vi "results graphing.vi"(0 "set to view":u32) -> (1 "N Meas":i32, 2 "Temperature":dbl, 3 "RC Fit":T4, 4 "RC Graph":waveform(dbl), 8 "results out":T3[](array[typedef]), 11 "N waves":i32 caption="Number of Waveforms", 12 "N done":i32 caption="Number Complete", 13 "meas":T1={"wvfm params"={"Num of avg"=100, "Num points"=1000, "Meas rate (Hz)"=100000.0}, "avg"={"t0"=timestamp(0 s since 1904-01-01), "dt"=1.0, "Y"=[]}, "raw wvfms"=[], "progress"={"avg done"=FALSE, "meas index"=0, "N waves"=0}, "t (s)"=0.0}, 14 "raw wvfms":waveform(dbl)[](array[waveform]), 15 "C vs T graph":cluster{dbl[], dbl[]})   [LabVIEW 2019]
doc: "This is a Bug C(T) subVI.\n\nIt extracts a variety of data from the results for presentation in the monitor loop.\n\nPaul K Dixon\nP3600\nCSUSB Physics"
uses:
  typedefs/result.ctl
  typedefs/cap fit params.ctl
  typedefs/measurement.ctl
  typedefs/wvfm acq params.ctl
  globals/Bug globals.vi
panel:
  out "result":T3={"Temp (C)"=0.0, "RC Fit"={"Resistance (Ohms)"=100000.0, "Est Time constant (s)"=0.0, "Est Capacitance (F)"=0.0}, "wave"={"t0"=timestamp(0 s since 1904-01-01), "dt"=1.0, "Y"=[]}, "Time (s)"=0.0}
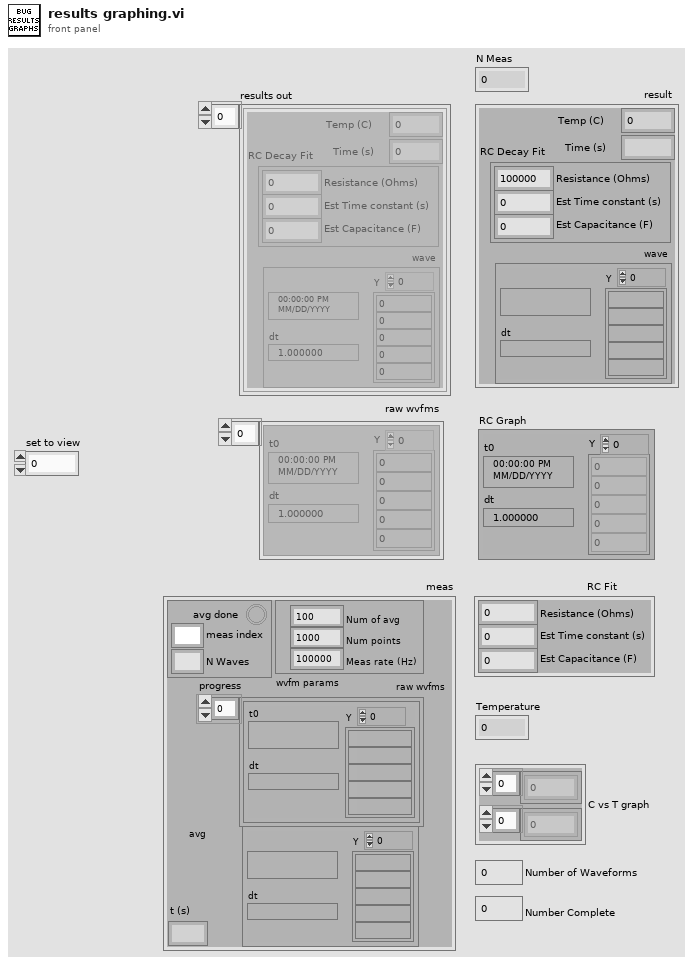
[diagram p1: front panel]
types:
  T1 = typedef "measurement.ctl" = cluster{"wvfm params":T2, "avg":waveform(dbl), "raw wvfms":waveform(dbl)[], "progress":cluster{"avg done":bool, "meas index":i32, "N waves":i32}, "t (s)":dbl}
  T2 = typedef "wvfm acq params.ctl" = cluster{"Num of avg":i32, "Num points":i32, "Meas rate (Hz)":dbl}
  T3 = typedef "result.ctl" = cluster{"Temp (C)":dbl, "RC Fit":T4, "wave":waveform(dbl), "Time (s)":dbl}
  T4 = typedef "cap fit params.ctl" = cluster{"Resistance (Ohms)":dbl, "Est Time constant (s)":dbl, "Est Capacitance (F)":dbl}
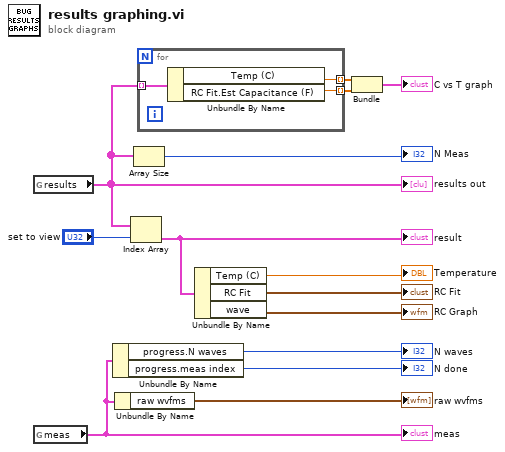
[diagram p0: block diagram]
diagram:
  n1 = global read "Bug globals.vi" "results"() -> (w5:T3[])
  "results out" <- w5
  n2 = global read "Bug globals.vi" "meas"() -> (w2:T1)
  "meas" <- w2
  n3 = Unbundle By Name(w2) -> ("progress.N waves"=→"N waves":i32, "progress.meas index"=→"N done":i32)
  n4 = Unbundle By Name(w2) -> ("raw wvfms"=→"raw wvfms":waveform(dbl)[])
  n5 = Index Array(array=w5, index="set to view") -> (element=w12:T3)
  "result" <- w12
  n6 = Array Size(array=w5) -> (size(s)=→"N Meas":i32)
  n7 = for {
    tunnel: w5 -> [w17] mode=indexing
    tunnel: [w16] -> w8 mode=indexing
    tunnel: [w15] -> w7 mode=indexing
    n8 = Unbundle By Name(w17) -> ("Temp (C)"=w16:dbl, "RC Fit.Est Capacitance (F)"=w15:dbl)
  }
  n9 = Unbundle By Name(w12) -> ("Temp (C)"=→"Temperature":dbl, "RC Fit"=→"RC Fit":T4, "wave"=→"RC Graph":waveform(dbl))
  n10 = Bundle(w8, w7) -> (→"C vs T graph":cluster{dbl[], dbl[]})  [unwired: 1 in]
